vi "add subresult.vi"(10 "subresult":refnum<class "result.lvclass">, 11 "result in":refnum<class "result.lvclass">) -> (3 "result out":refnum<class "result.lvclass">)   [LabVIEW 2013, in "result.lvclass"]
uses:
  result.lvclass
  result.lvclass/result.ctl
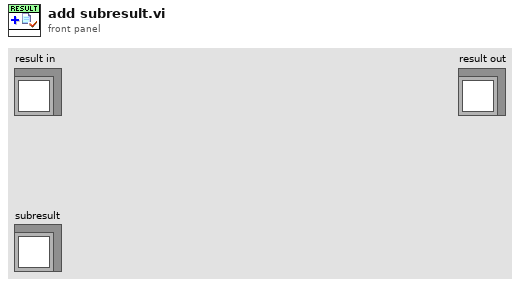
[diagram p1: front panel]
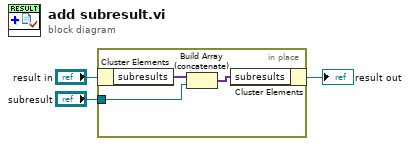
[diagram p0: block diagram]
diagram:
  n1 = in-place {
    in-place-border: "subresult" -> [w4]
    n2 = in-place-cluster #1("result in") -> ("subresults"=w6:variant[])
    n3 = Build Array (concatenate)(w6, w4) -> (w5:variant[])
    n4 = in-place-cluster #1("subresults"=w5) -> (→"result out":refnum<class "result.lvclass">)
  }
